vi "Register Remove Team Event.vi"(8 "error in (no error)":errorcluster, 10 "Remove Team":refnum<user-event>, 11 "Game Config Panel in":refnum<class "Game Config Panel.lvclass">) -> (0 "error out":errorcluster, 3 "Game Config Panel out":refnum<class "Game Config Panel.lvclass">)   [LabVIEW 2020, in "SB App.lvlib" / "Game Config Panel.lvclass"]
uses:
  Game Config Panel.lvclass
  SquareBattle/Team ID.ctl
  Game Config Panel.lvclass/Game Config Panel.ctl
  SquareBattle/SquareBattle.lvlib
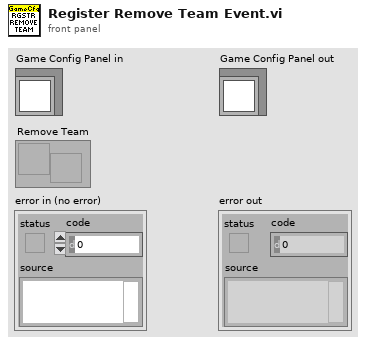
[diagram p1: front panel]
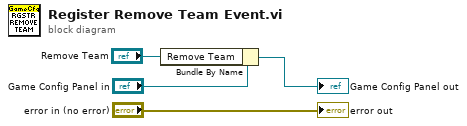
[diagram p0: block diagram]
diagram:
  n1 = Bundle By Name(cluster="Game Config Panel in", "Remove Team"="Remove Team") -> (→"Game Config Panel out":refnum<class "Game Config Panel.lvclass">)
  "error out" <- "error in (no error)"
